vi "Galvo_track.vi"(4 "Samples per channel":i32, 5 "Sample rate (Hz)":dbl, 7 "error in (no error)":errorcluster, 10 "Samp Clk. Delay Units":i32(ring)=10364 items=["Seconds"=10364, "Ticks"=10304], 11 "Sample Clock Delay":dbl, 14 "Sample clock source":tag="/Dev1/PFI0", 17 "Delay from sample clock":bool) -> (20 "task out":refnum<k21>, 27 "error out":errorcluster)   [LabVIEW 2014]
uses:
  <vilib>/DAQmx/create/channels.llb/DAQmx Create Channel (AI-Voltage-Basic).vi
  <vilib>/DAQmx/read.llb/DAQmx Read.vi
  <vilib>/DAQmx/read.llb/DAQmx Read (Analog 1D Wfm NChan NSamp).vi
  <vilib>/DAQmx/configure/timing.llb/DAQmx Timing (Sample Clock).vi
  <resource>/objmgr/daqmx.rc
panel:
  in  "Sample Clock Delay 3":dbl
  out "data":waveform(dbl)[](graph)
  in  "Sample Clock Delay 2":dbl
  in  "Z axis":T1
  in  "Slow axis":T1
  in  "Fast axis":T1
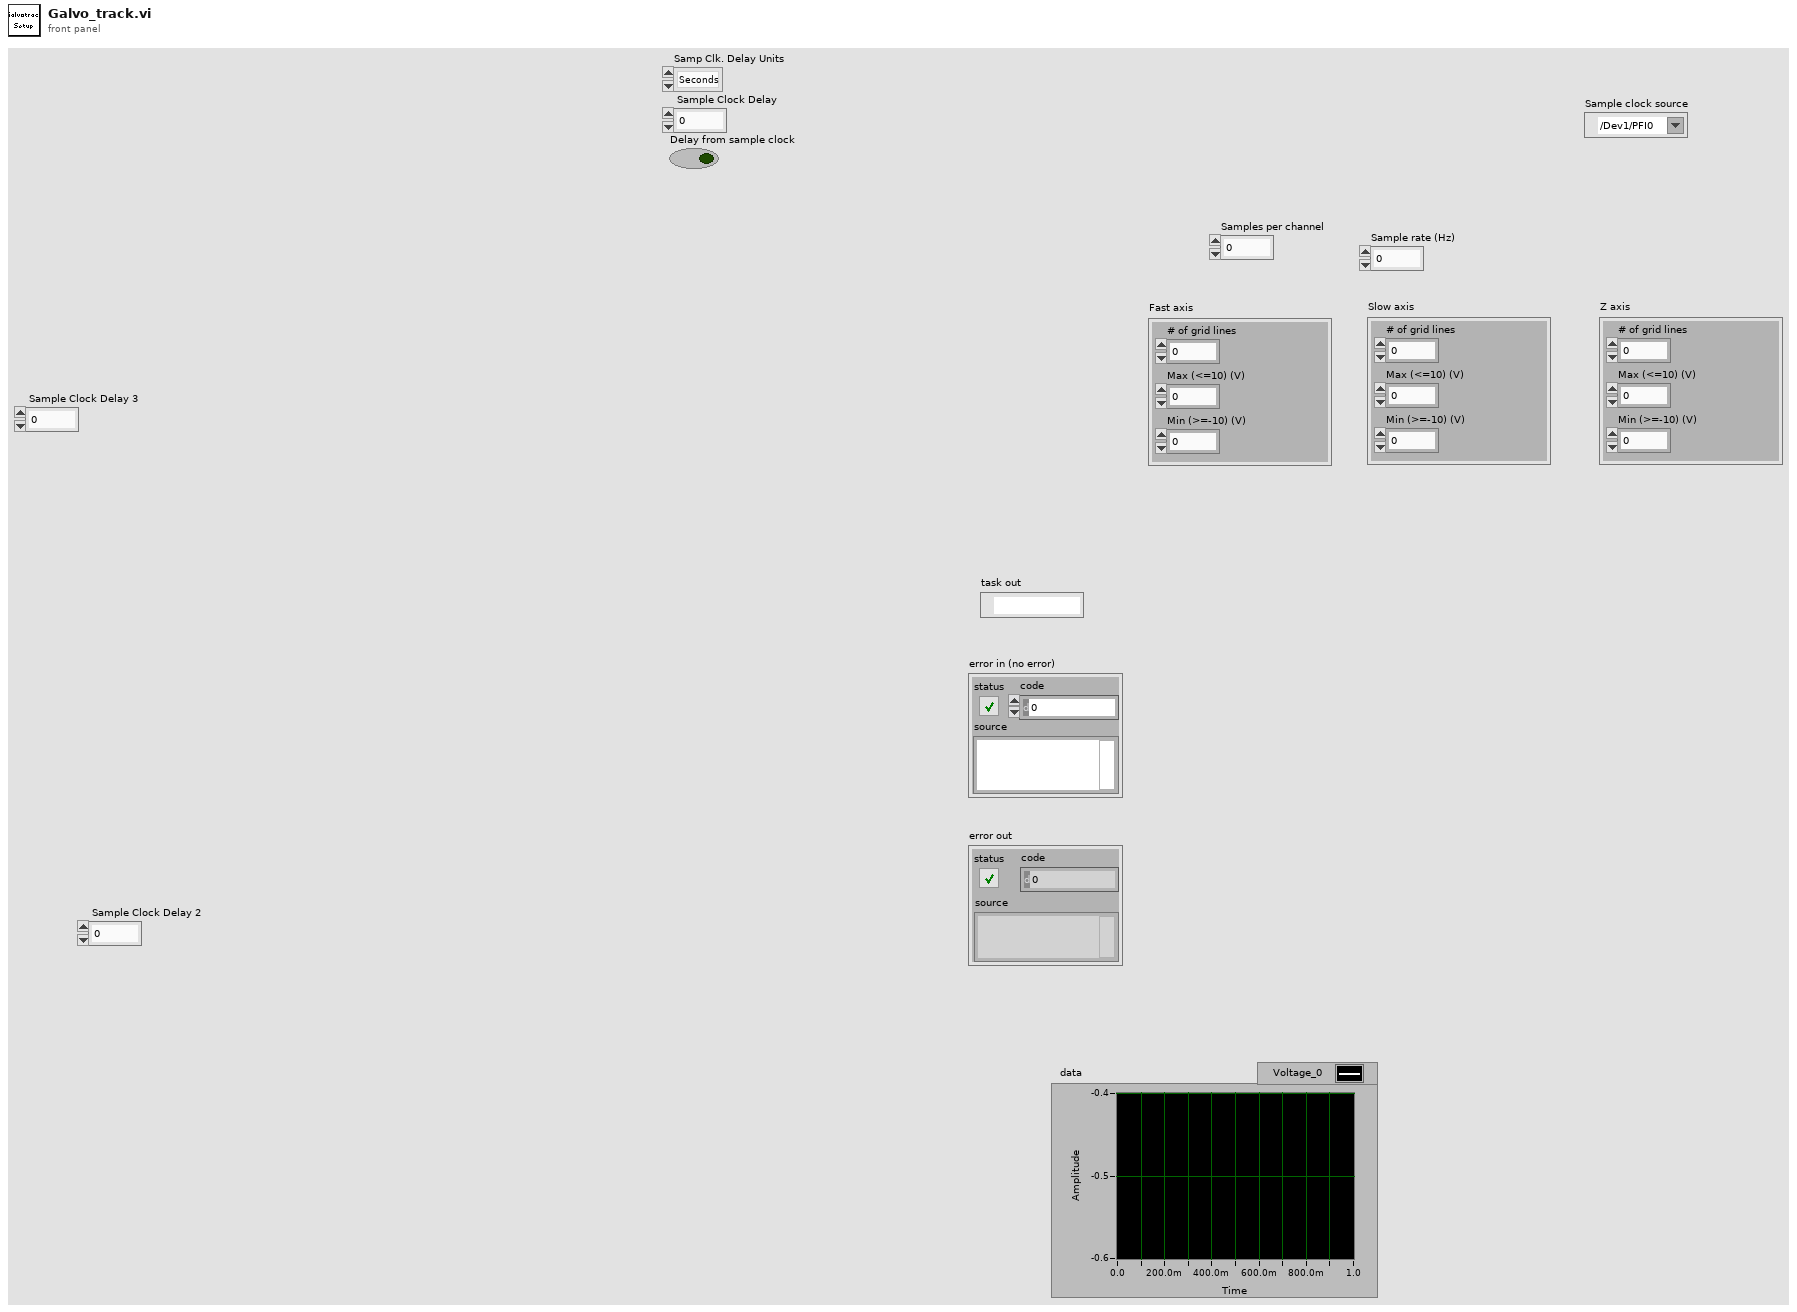
[diagram p1: front panel]
types:
  T1 = cluster{"# of grid lines":u16, "Max (<=10) (V)":dbl, "Min (>=-10) (V)":dbl}
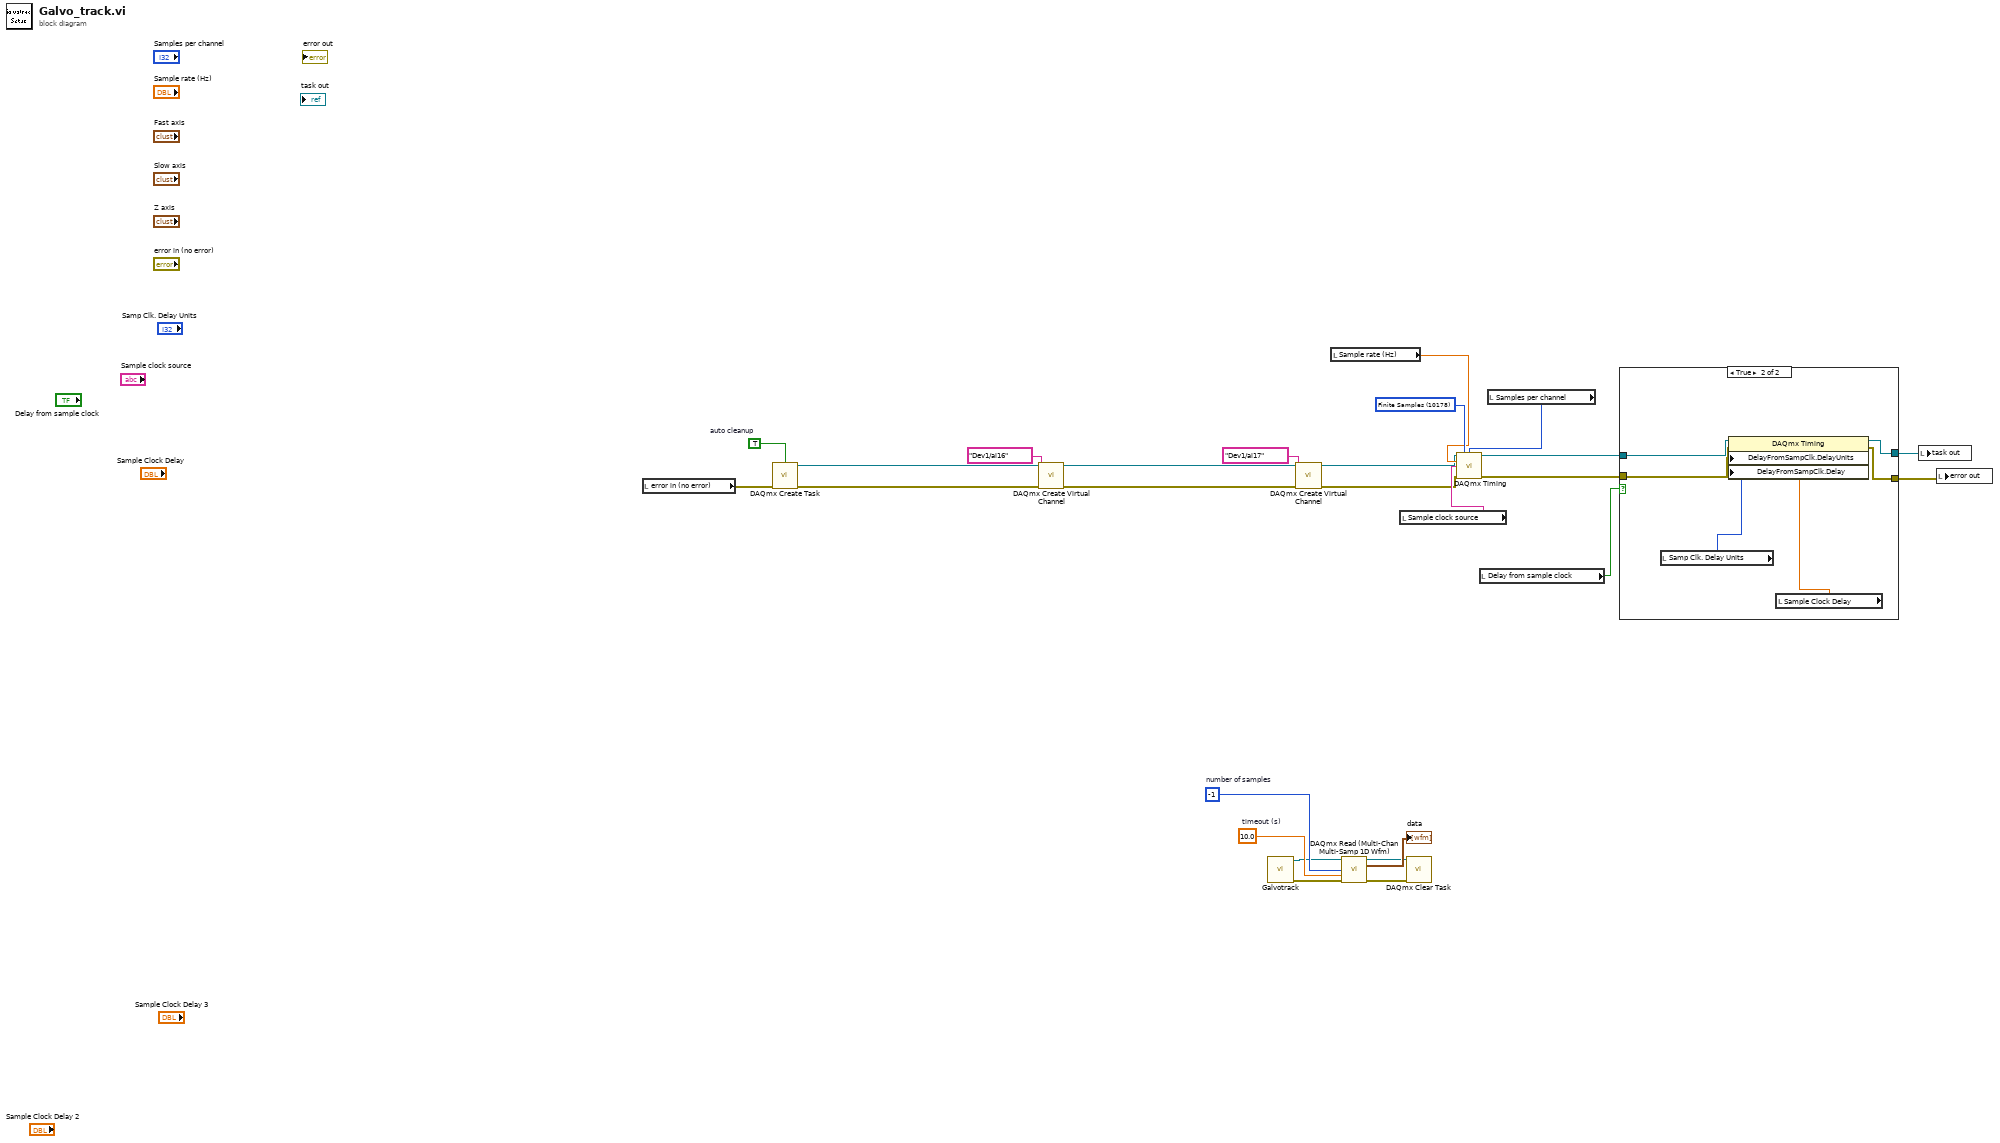
[diagram p0: block diagram]
diagram:
  w11 = 10178 items=["Finite Samples"=10178, "Continuous Samples"=10123, "Hardware Timed Single Point"=12522] ("sample mode")
  w18 = TRUE  # auto cleanup
  w24 = 10.0  # timeout (s)
  w25 = -1  # number of samples
  n1 = local read "error in (no error)"() -> (w12:errorcluster)
  n2 = call <vilib>:"DAQmx Create Task.vi"("auto cleanup"=w18, "error in"=w12) -> ("task out"=w17:refnum<k21>, "error out"=w19:errorcluster)  [unwired: 12 in]
  n3 = call-poly <vilib>:"DAQmx Create Virtual Channel.vi"("task in"=w17, "physical channels"=tag "Dev1/ai16", "error in"=w19) -> ("task out"=w15:refnum<k21>, "error out"=w16:errorcluster)  [unwired: 11 in]
  n4 = call "Galvotrack.vi"() -> ("error out"=w20:errorcluster, "task out"=w21:refnum<k21>)  [unwired: 10 in]
  n5 = call-poly <vilib>:"DAQmx Create Virtual Channel.vi"("task in"=w15, "physical channels"=tag "Dev1/ai17", "error in"=w16) -> ("task out"=w2:refnum<k21>, "error out"=w1:errorcluster)  [unwired: 11 in]
  n6 = local read "Sample rate (Hz)"() -> (w4:dbl)
  n7 = call-poly "DAQmx Read (Multi-Chan Multi-Samp 1D Wfm).vi"("task/channels in"=w21, "number of samples per channel"=w25, "timeout"=w24, "error in"=w20) -> ("task out"=w22:refnum<k21>, "data"=→"data":waveform(dbl)[], "error out"=w23:errorcluster)  [unwired: 9 in]
  n8 = local read "Sample clock source"() -> (w9:tag)
  n9 = call <vilib>:"DAQmx Clear Task.vi"("task in"=w22, "error in"=w23) -> ()  [unwired: 13 in, 1 out]
  n10 = local read "Delay from sample clock"() -> (w3:bool)
  n11 = local read "Samples per channel"() -> (w10:i32)
  n12 = call-poly <vilib>:"DAQmx Timing.vi"("task/channels in"=w2, "sample mode"=w11, "samples per channel"=w10, "rate"=w4, "source"=w9, "error in"=w1) -> ("task out"=w6:refnum<k21>, "error out"=w5:errorcluster)  [unwired: 8 in]
  n13 = case shown="True" w3 {
    tunnel: [w28 w34] -> w8
    tunnel: [w27 w33] -> w7
    tunnel: w6 -> [w28 w32]
    tunnel: w5 -> [w27 w31]
    frame False {
    }
    frame True {
      n14 = local read "Samp Clk. Delay Units"() -> (w29:i32)
      n15 = local read "Sample Clock Delay"() -> (w30:dbl)
      n16 = property class="DAQmx Timing"(reference=w32, error in=w31, "DelayFromSampClk.DelayUnits"=w29, "DelayFromSampClk.Delay"=w30) -> (reference out=w34:refnum<k21>, error out=w33:errorcluster)
    }
  }
  n17 = local write "task out"(w8) -> ()
  n18 = local write "error out"(w7) -> ()
